vi "ShoreDefinition.vi"(0 "Image In":T1, 7 "error in":errorcluster) -> (20 "Image Out":T1, 27 "error out":errorcluster)   [LabVIEW 2014]
uses:
  <vilib>/vision/Image Controls.llb/IMAQ Image.ctl
  <vilib>/vision/NI_Vision_Development_Module.lvlib
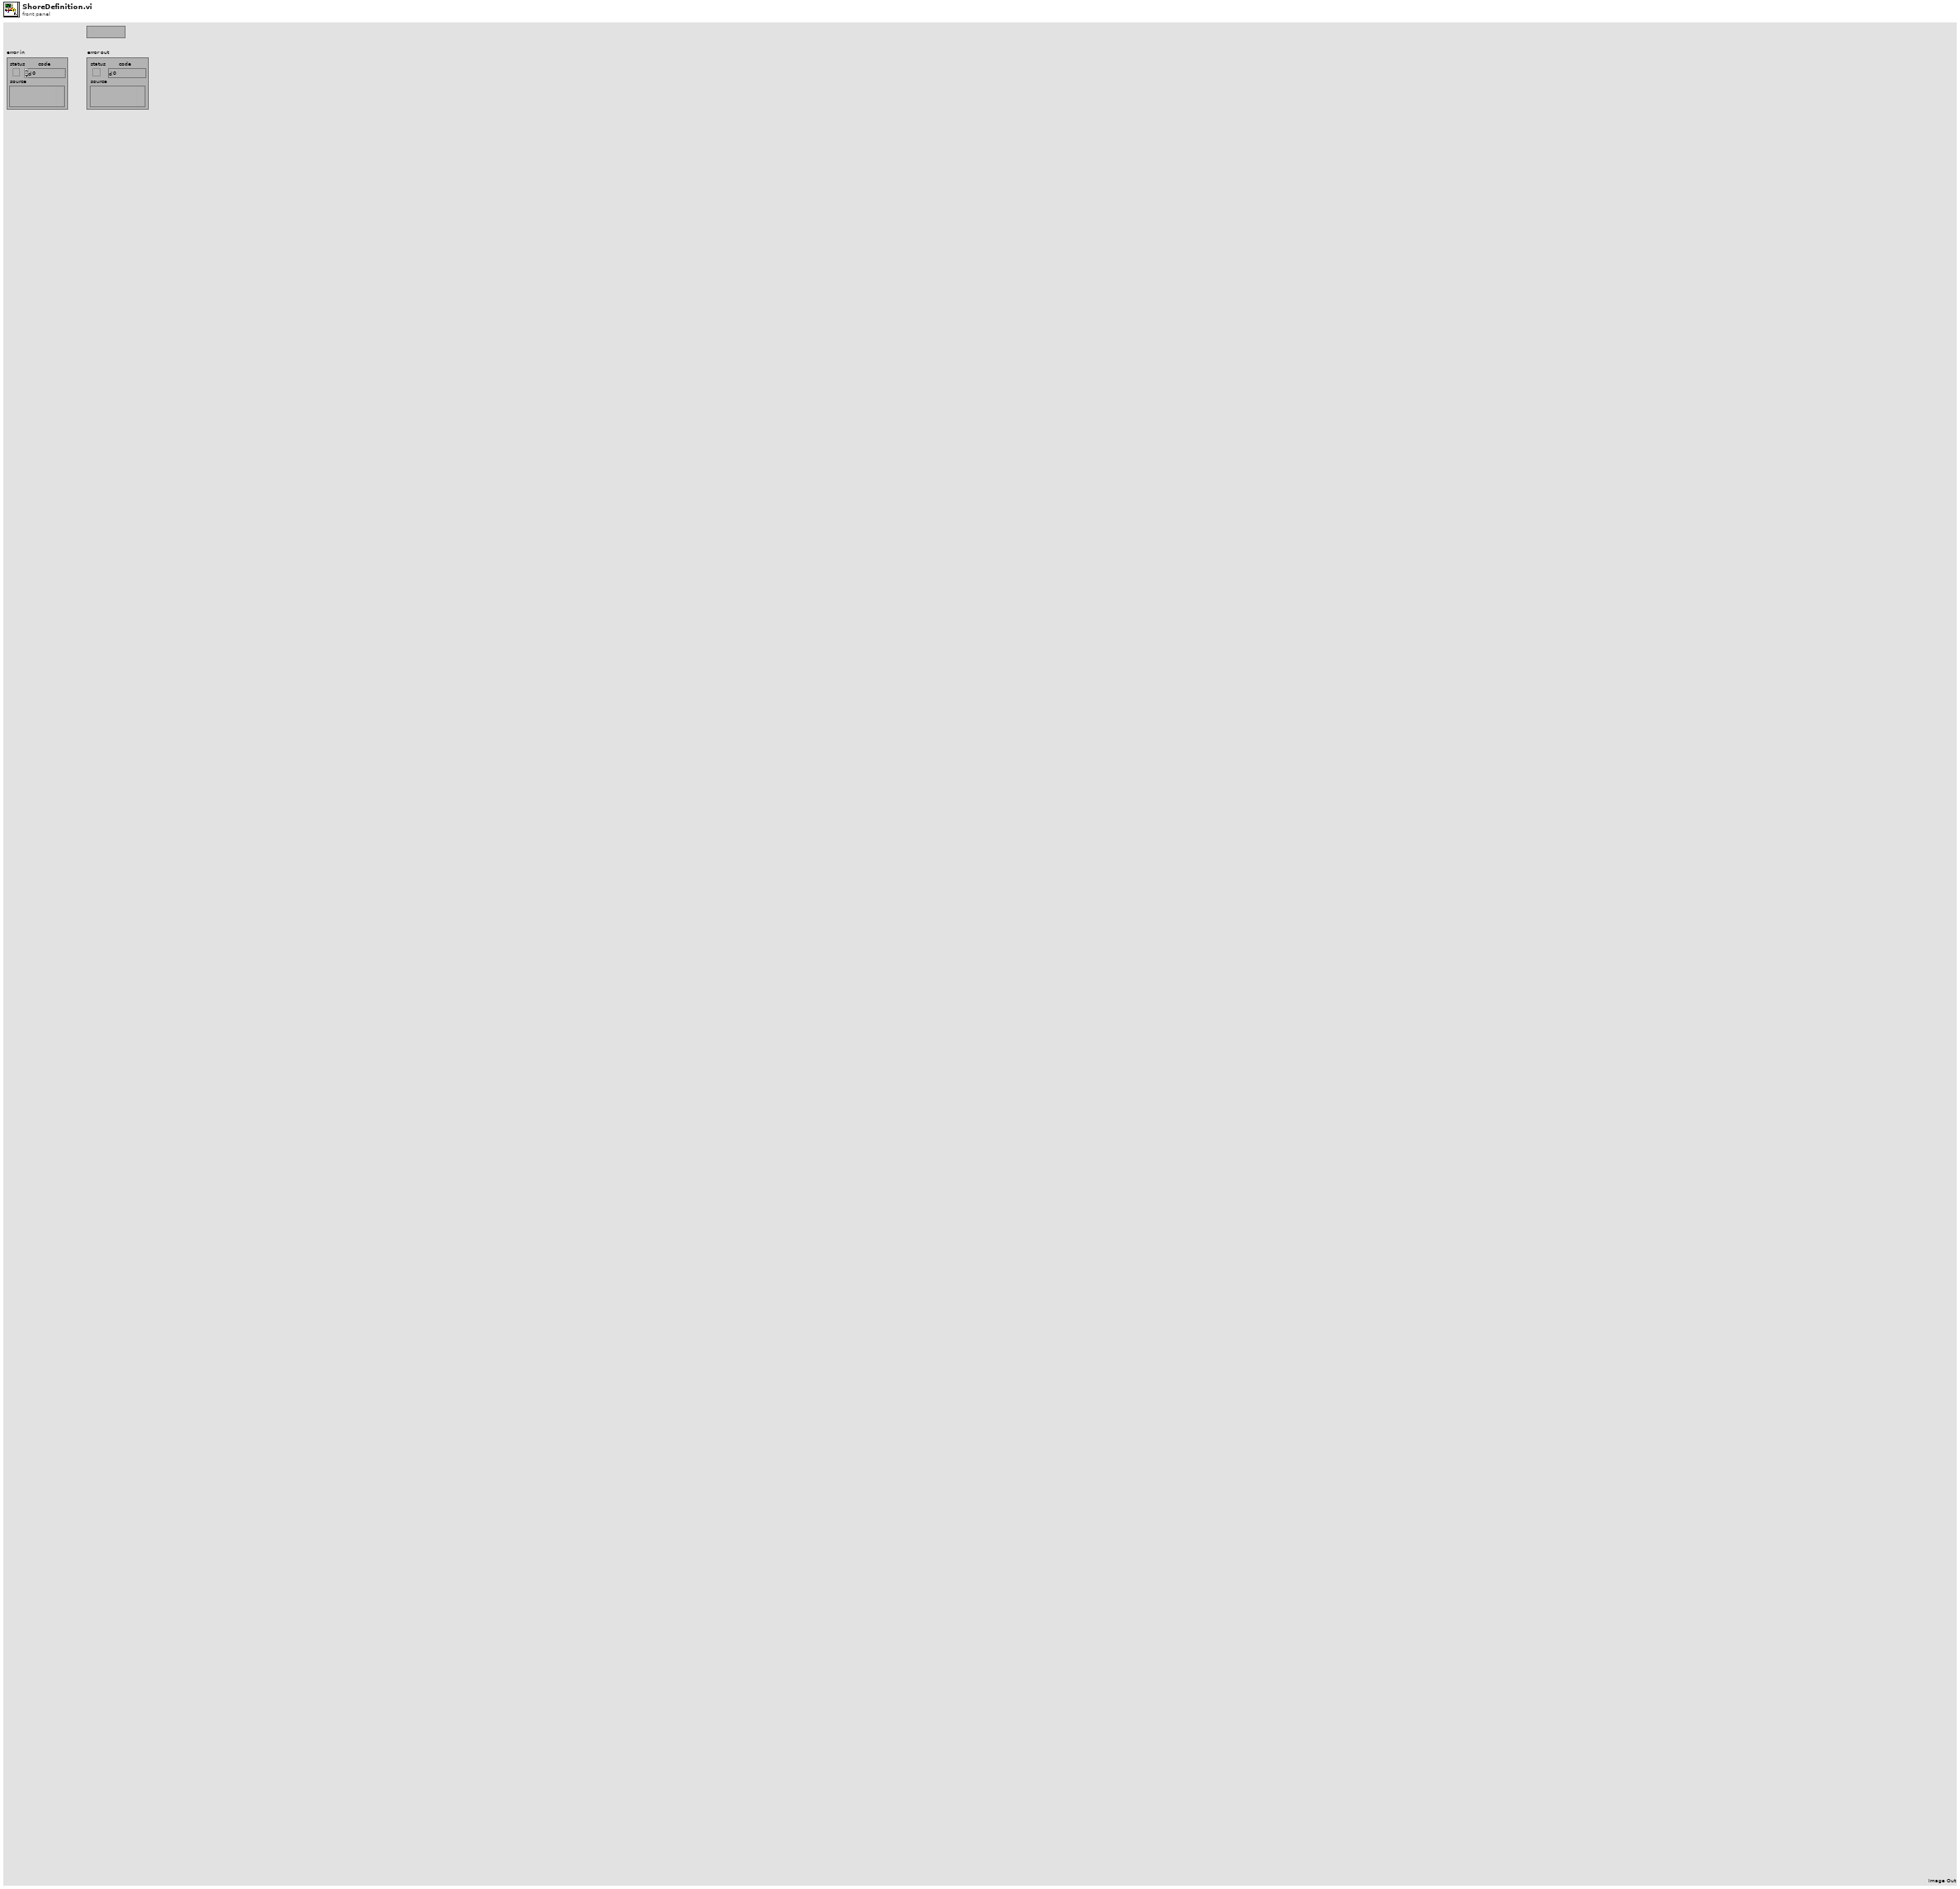
[diagram p1: front panel]
types:
  T1 = typedef "IMAQ Image.ctl" = refnum<image>
  T2 = enum32{"AutoM", "Close", "Dilate", "Erode", "Gradient", "Gradient out", "Gradient in", "Hit miss", "Open", "PClose", "POpen", "Thick", "Thin"}
  T3 = typedef "Image Type" = u32
  T4 = cluster{"Brightness":sgl, "Contrast":sgl, "Gamma":sgl}
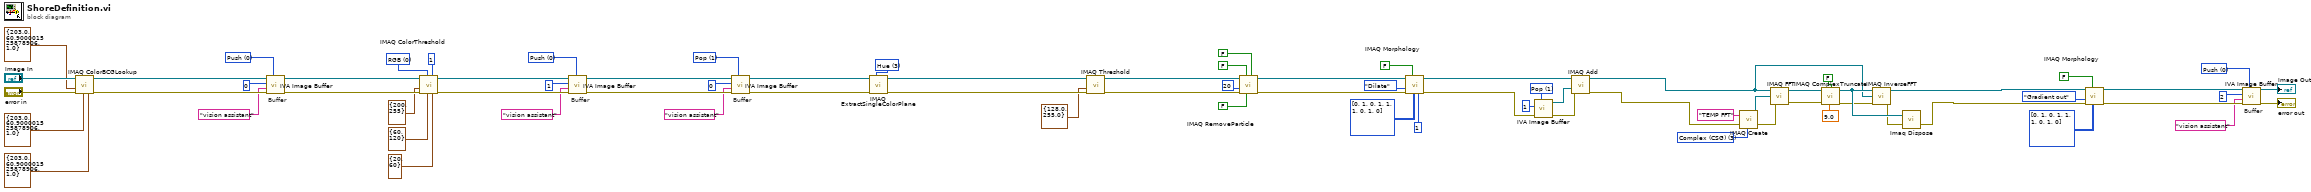
[diagram p0: block diagram]
diagram:
  w4 = u16 0 items=["Push", "Pop", "Reset"] ("Function")
  w12 = T3 3 items=["Grayscale (U8)", "Grayscale (I16)", "Grayscale (SGL)", "Complex (CSG)", "RGB (U32)", "HSL (U32)", "RGB (U64)", "Grayscale (U16)"] ("Image Type")
  w30 = u16 1 items=["Push", "Pop", "Reset"] ("Function")
  w48 = 3 items=["Red", "Green", "Blue", "Hue", "Saturation", "Luminance", "Value", "Intensity"] ("Color Plane")
  w51 = u16 1 items=["Push", "Pop", "Reset"] ("Function")
  w56 = u16 0 items=["Push", "Pop", "Reset"] ("Function")
  w64 = u16 0 items=["RGB", "HSL", "HSV", "HSI"] ("Color Mode")
  w68 = u16 0 items=["Push", "Pop", "Reset"] ("Function")
  # "Buffer"
  # "Buffer"
  # "Buffer"
  # "Buffer"
  n1 = call "IMAQ ColorBCGLookup"("Blue BCG Values"=T4 {"Brightness"=203.0, "Contrast"=60.9, "Gamma"=1.0}, "Green BCG Values"=T4 {"Brightness"=203.0, "Contrast"=60.9, "Gamma"=1.0}, "error in (no error)"="error in", "Red BCG Values"=T4 {"Brightness"=203.0, "Contrast"=60.9, "Gamma"=1.0}, "Image Src"="Image In") -> ("error out"=w74:errorcluster, "Image Dst Out"=w70:T1)  [unwired: 2 in, 3 out]
  n2 = call <vilib>:"IVA Image Buffer.vi"("Function"=w68, "error in (no error)"=w74, "Prefix"="vision assistant", "Buffer #"=0, "Image In"=w70) -> ("error out"=w69:errorcluster, "Image Out"=w60:T1)  [unwired: 5 out]
  n3 = call "IMAQ ColorThreshold"("Blue or Luma or Val or Inten Range"=cluster{"Lower value":i32, "Upper value":i32} {"Lower value"=20, "Upper value"=60}, "Replace Value"=1, "Green or Sat Range"=cluster{"Lower value":i32, "Upper value":i32} {"Lower value"=60, "Upper value"=120}, "Color Mode"=w64, "error in (no error)"=w69, "Red or Hue Range"=cluster{"Lower value":i32, "Upper value":i32} {"Lower value"=200, "Upper value"=255}, "Image Src"=w60) -> ("error out"=w59:errorcluster, "Image Dst Out"=w58:T1)  [unwired: 1 in, 2 out]
  n4 = call <vilib>:"IVA Image Buffer.vi"("Function"=w56, "error in (no error)"=w59, "Prefix"="vision assistant", "Buffer #"=1, "Image In"=w58) -> ("error out"=w57:errorcluster, "Image Out"=w53:T1)  [unwired: 5 out]
  n5 = call <vilib>:"IVA Image Buffer.vi"("Function"=w51, "error in (no error)"=w57, "Prefix"="vision assistant", "Buffer #"=0, "Image In"=w53) -> ("error out"=w52:errorcluster, "Image Out"=w47:T1)  [unwired: 5 out]
  n6 = call "IMAQ ExtractSingleColorPlane"("Color Plane"=w48, "error in (no error)"=w52, "Image Src"=w47) -> ("error out"=w46:errorcluster, "Image Dst Out"=w44:T1)  [unwired: 1 in, 6 out]
  n7 = call "IMAQ Threshold"("error in (no error)"=w46, "Range"=cluster{"Lower value":sgl, "Upper value":sgl} {"Lower value"=128.0, "Upper value"=255.0}, "Image Src"=w44) -> ("error out"=w43:errorcluster, "Image Dst Out"=w38:T1)  [unwired: 3 in, 4 out]
  n8 = call "IMAQ RemoveParticle"("Connectivity 4/8 (8)"=FALSE, "Low Pass/High Pass (Low)"=FALSE, "Square/Hexa (Square)"=FALSE, "error in (no error)"=w43, "Number of Erosion"=20, "Image Src"=w38) -> ("error out"=w37:errorcluster, "Image Dst Out"=w32:T1)  [unwired: 1 in, 3 out]
  n9 = call "IMAQ Morphology"("Number of iterations (1)"=1, "Structuring Element"=i32[][] [[0, 1, 0], [1, 1, 1], [0, 1, 0]], "Square/Hexa (Square)"=FALSE, "error in (no error)"=w37, "Operation"=T2."Dilate", "Image Src"=w32) -> ("error out"=w31:errorcluster, "Image Dst Out"=w27:T1)  [unwired: 1 in, 3 out]
  n10 = call <vilib>:"IVA Image Buffer.vi"("Function"=w30, "error in (no error)"=w31, "Buffer #"=1) -> ("error out"=w26:errorcluster, "Image Out"=w28:T1)  [unwired: 2 in, 5 out]
  n11 = call "IMAQ Add"("Image Src A"=w27, "Image Src B"=w28, "error in (no error)"=w26) -> ("Image Dst Out"=w15:T1, "error out"=w25:errorcluster)  [unwired: 2 in, 2 out]
  n12 = call "IMAQ Create"("Image Name"="TEMP FFT", "Image Type"=w12, "error in (no error)"=w25) -> ("New Image"=w23:T1, "error out"=w16:errorcluster)  [unwired: 1 in, 1 out]
  n13 = call "IMAQ FFT"("error in (no error)"=w16, "Image Dst"=w23, "Image Src"=w15) -> ("error out"=w21:errorcluster, "Image Dst Out"=w22:T1)  [unwired: 1 out]
  n14 = call "IMAQ ComplexTruncate"("error in (no error)"=w21, "Truncation Frequency %"=sgl 9.0, "Image Src"=w22, "Low pass/High pass (Low pass)"=FALSE) -> ("error out"=w19:errorcluster, "Image Dst Out"=w20:T1)  [unwired: 1 in, 2 out]
  n15 = call "IMAQ InverseFFT"("error in (no error)"=w19, "Image Dst"=w15, "Image Src"=w20) -> ("error out"=w18:errorcluster, "Image Dst Out"=w8:T1)  [unwired: 1 out]
  n16 = call "Imaq Dispose"("Image"=w20, "error in (no error)"=w18) -> ("error out"=w17:errorcluster)  [unwired: 1 in, 3 out]
  n17 = call "IMAQ Morphology"("Structuring Element"=i32[][] [[0, 1, 0], [1, 1, 1], [0, 1, 0]], "Square/Hexa (Square)"=FALSE, "error in (no error)"=w17, "Operation"=T2."Gradient out", "Image Src"=w8) -> ("error out"=w7:errorcluster, "Image Dst Out"=w6:T1)  [unwired: 2 in, 3 out]
  n18 = call <vilib>:"IVA Image Buffer.vi"("Function"=w4, "error in (no error)"=w7, "Prefix"="vision assistant", "Buffer #"=2, "Image In"=w6) -> ("error out"=→"error out":errorcluster, "Image Out"=→"Image Out":T1)  [unwired: 5 out]
